vi "runScript.vi"(8 "error in (no error)":errorcluster, 10 "Path":path, 11 "CompiledList in":refnum<class "CompiledList.lvclass">) -> (0 "error out":errorcluster, 1 "Path out":path, 2 "CompiledScript":T1, 3 "CompiledList out":refnum<class "CompiledList.lvclass">, 4 "found?":bool, 5 "TimeStamp":string)   [LabVIEW 2009, in "Compiler.lvlib" / "CompiledList.lvclass"]
uses:
  CompiledList.lvclass
  ScriptListCompiler/ScriptListCompiler.lvclass
  Hal/Channels/VoltOutput/AnalogOutput.lvclass
  Hal/Channels/Digital/DigitalOutput.lvclass
  Hal/Channels/DDSOutput/Generic/DDSOutput.lvclass
  Filing/FileNeologist/FileNeologist.lvclass
  Filing.lvlib
  Compiler.lvlib
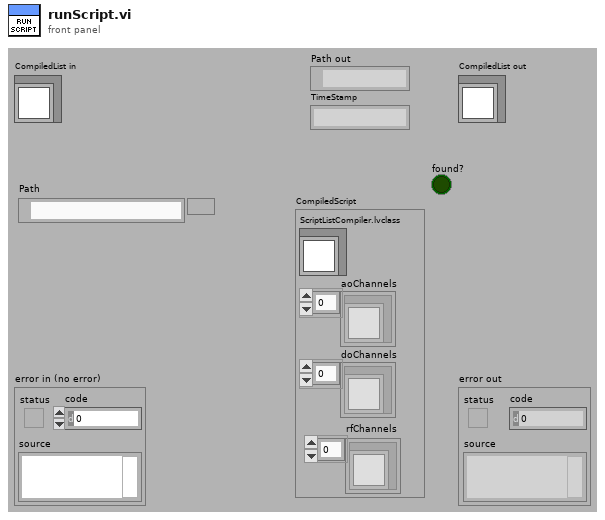
[diagram p1: front panel]
types:
  T1 = cluster{"ScriptListCompiler.lvclass":refnum<class "ScriptListCompiler.lvclass">, "aoChannels":refnum<class "AnalogOutput.lvclass">[], "doChannels":refnum<class "DigitalOutput.lvclass">[], "rfChannels":refnum<class "DDSOutput.lvclass">[]}
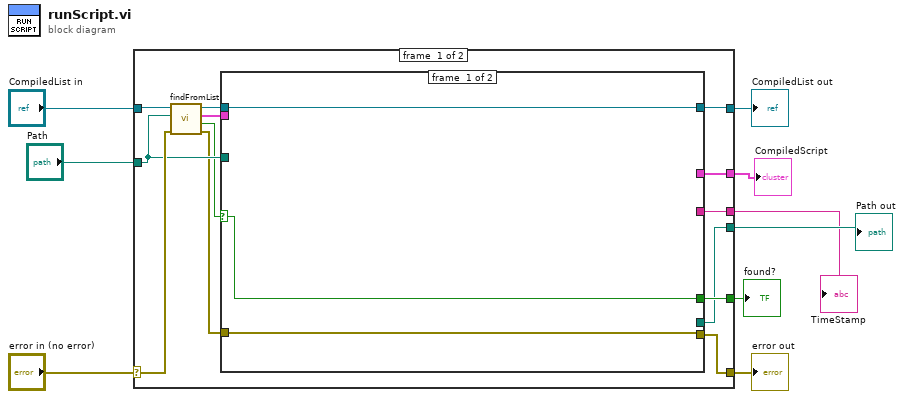
[diagram p0: block diagram]
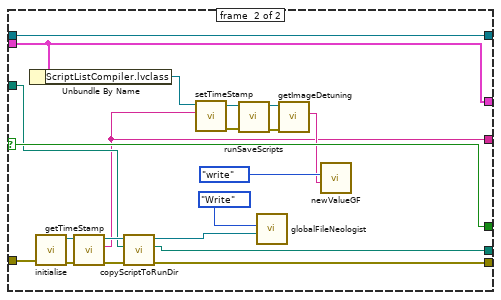
[diagram p2: hidden frame]
diagram:
  n1 = case shown="No Error" "error in (no error)" {
    selector: "error in (no error)" -> [w21 w48]
    tunnel: [w14 w48] -> w8
    tunnel: [w15 w47] -> w6
    tunnel: "CompiledList in" -> [w22 w47]
    tunnel: "Path" -> [w20 _]
    tunnel: [w13 _] -> w4
    tunnel: [w12 _] -> w3
    tunnel: [w11 _] -> w2
    tunnel: [w10 _] -> w1
    frame #0 {
      n2 = call "findFromList.vi"("error in (no error)"=w21, "Path"=w20, "CompiledList in"=w22) -> ("error out"=w17:errorcluster, "found?"=w18:bool, "CompiledScript"=w19:T1, "CompiledList out"=w16:refnum<class "CompiledList.lvclass">)  [unwired: 5 in]
      n3 = case shown="True" w18 {
        selector: w18 -> [w23 w36]
        tunnel: w20 -> [_ w31]
        tunnel: w19 -> [_ w30]
        tunnel: w17 -> [w24 w41]
        tunnel: w16 -> [w25 w37]
        tunnel: [w25 w37] -> w15
        tunnel: [w24 w28] -> w14
        tunnel: [w23 w36] -> w13
        tunnel: [_ w30] -> w12
        tunnel: [_ w27] -> w11
        tunnel: [_ w26] -> w10
        frame #0 {
        }
        frame #1 {
          n4 = Unbundle By Name(w30) -> ("ScriptListCompiler.lvclass"=w40:refnum<class "ScriptListCompiler.lvclass">)
          n5 = call "initialise.vi"("error in (no error)"=w41) -> ("error out"=w45:errorcluster, "FileNeologist out"=w46:refnum<class "FileNeologist.lvclass">)  [unwired: 9 in]
          n6 = call "getTimeStamp.vi"("error in (no error)"=w45, "FileNeologist in"=w46) -> ("error out"=w42:errorcluster, "TimeStamp"=w26:string, "FileNeologist out"=w43:refnum<class "FileNeologist.lvclass">)  [unwired: 7 in]
          n7 = call-dynamic "copyScriptToRunDir.vi"("error in (no error)"=w42, "Path in"=w31, "FileNeologist in"=w43) -> ("error out"=w28:errorcluster, "Path out"=w27:path, "FileNeologist out"=w29:refnum<class "FileNeologist.lvclass">)  [unwired: 6 in]
          n8 = call "setTimeStamp.vi"("timeStamp"=w26, "ScriptListCompiler in"=w40) -> ("error out"=w38:errorcluster, "ScriptListCompiler out"=w39:refnum<class "ScriptListCompiler.lvclass">)  [unwired: 8 in]
          n9 = call "runSaveScripts.vi"("error in (no error)"=w38, "ScriptListCompiler in"=w39) -> ("error out"=w34:errorcluster, "ScriptListCompiler out"=w35:refnum<class "ScriptListCompiler.lvclass">)  [unwired: 8 in]
          n10 = call "globalFileNeologist.vi"("FileNeologist in"=w29, "Action"=enum16{"Write", "Read"}."Write") -> ()  [unwired: 9 in, 1 out]
          n11 = call "getImageDetuning.vi"("error in (no error)"=w34, "ScriptListCompiler in"=w35) -> ("ImageDetuning"=w32:string)  [unwired: 7 in, 2 out]
          n12 = call "newValueGF.vi"("newValue"=w32, "control"=enum16{"read", "write"}."write") -> ()  [unwired: 9 in, 1 out]
        }
      }
    }
    frame #1 {
    }
  }
  "error out" <- w8
  "CompiledList out" <- w6
  "found?" <- w4
  "CompiledScript" <- w3
  "Path out" <- w2
  "TimeStamp" <- w1
